vi "Handler_Add Proxy.vi"(4 "PreAuthenticate":bool, 6 "UseProxy":bool, 8 "error in (no error)":errorcluster, 10 "WebProxy":refnum<class "WebProxy_NET.lvclass">, 11 "LabVIEWHTTPClient_NET in":refnum<class "HttpClient_NET.lvclass">) -> (0 "error out":errorcluster, 3 "LabVIEWHTTPClient_NET out":refnum<class "HttpClient_NET.lvclass">)   [LabVIEW 2018, in "HttpClient_NET.lvlib" / "HttpClient_NET.lvclass"]
doc: "<b> </b> <b> </b>\nHttpClient_NET\nJustin Young - Viviota\nCopyright (c) 2021\nLicense: BSD"
uses:
  HttpClient_NET.lvclass
  WebProxy_NET/WebProxy_NET.lvclass
  HttpClient_NET.lvclass/HttpClient_NET.ctl
  WebProxy_NET/WebProxy_NET.lvclass/WebProxy_NET.ctl
  System.Net.Http
  Accessors/Read NET_HttpClientHandler.vi
  WebProxy_NET/Accessors/Read NET_WebProxy.vi
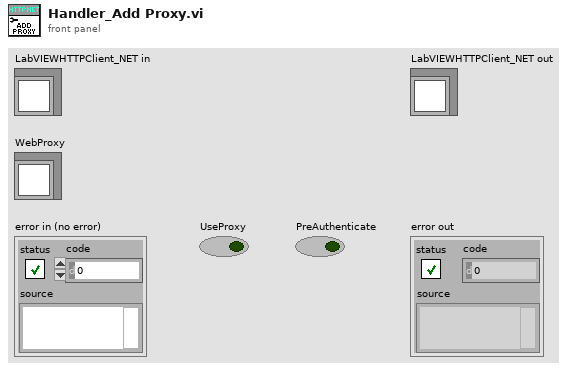
[diagram p1: front panel]
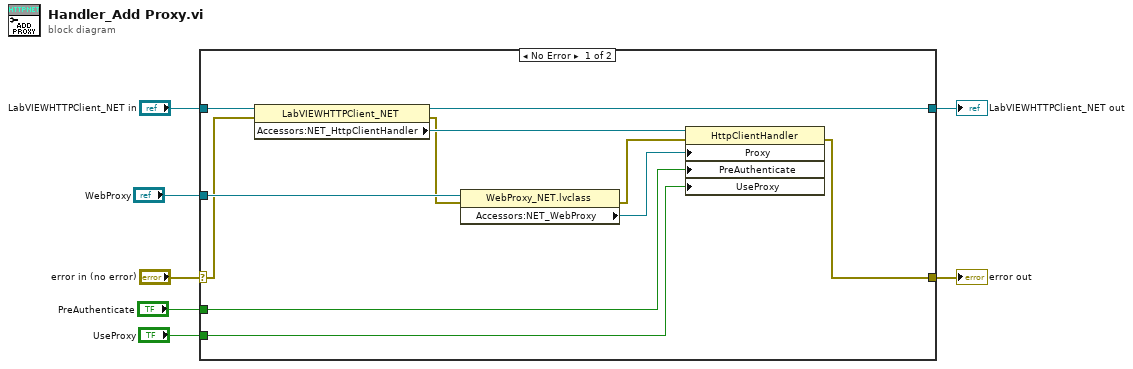
[diagram p0: block diagram]
diagram:
  n1 = case shown="No Error" "error in (no error)" {
    selector: "error in (no error)" -> [w11 w20]
    tunnel: [w8 w20] -> w6
    tunnel: [w17 w19] -> w4
    tunnel: "LabVIEWHTTPClient_NET in" -> [w18 w19]
    tunnel: "WebProxy" -> [w16 _]
    tunnel: "UseProxy" -> [w13 _]
    tunnel: "PreAuthenticate" -> [w12 _]
    frame No Error {
      n2 = property class="LabVIEWHTTPClient_NET"(reference=w18, error in=w11) -> (reference out=w17:refnum<class "HttpClient_NET.lvclass">, error out=w10:errorcluster, "Accessors:NET_HttpClientHandler"=w15:refnum<k24>)
      n3 = property class="WebProxy_NET.lvclass"(reference=w16, error in=w10) -> (error out=w9:errorcluster, "Accessors:NET_WebProxy"=w14:refnum<k24>)  [unwired: 1 out]
      n4 = property class="HttpClientHandler"(reference=w15, error in=w9, "Proxy"=w14, "PreAuthenticate"=w12, "UseProxy"=w13) -> (error out=w8:errorcluster)  [unwired: 1 out]
    }
    frame Error {
    }
  }
  "error out" <- w6
  "LabVIEWHTTPClient_NET out" <- w4
